vi "AlmacenamientoDatos.vi"(2 "array":dbl[](array[numeric])) -> ()   [LabVIEW 2014]
doc: "Demonstrates how to create a .xlsx file with the Write To Measurement File Express VI. A .xlsx file can be opened in Microsoft Excel 2007 or later. Running this example does not require Microsoft Excel to be installed on this computer."
panel:
  out "appended array":dbl[](array[numeric])
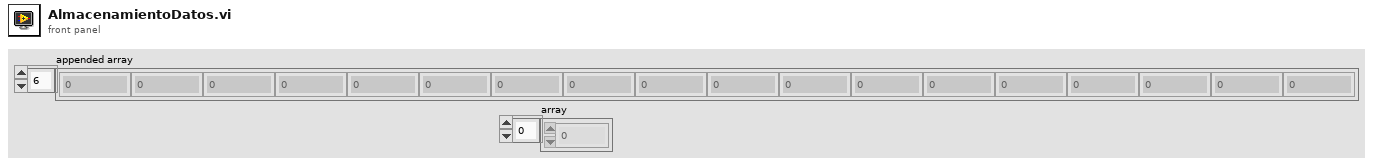
[diagram p1: front panel]
types:
  T1 = enum16{"big-endian, network order", "native, host order", "little-endian"}
  T2 = enum16{"open", "replace", "create", "open or create", "replace or create", "replace or create with confirmation"}
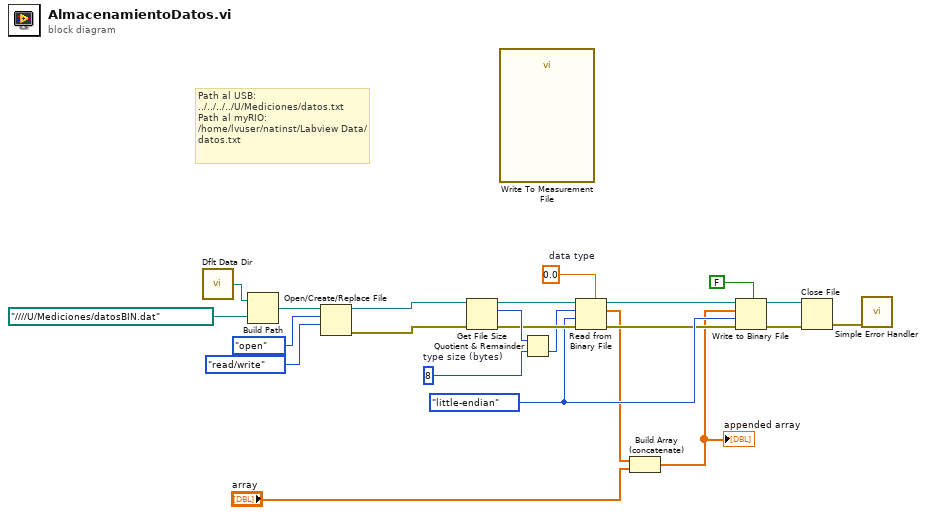
[diagram p0: block diagram]
diagram:
  w4 = 0.0  # data type
  w11 = i64 8  # type size (bytes)
  w8 = T1."little-endian" ("byte order (0:big-endian, network order)")
  # "Path al USB:\n../../../../U/Mediciones/datos.txt\nPath al myRIO:\n/home/lvuser/natinst/Labview Data/datos.txt"
  n1 = call <vilib>:"Dflt Data Dir.vi"() -> ("App:Default Data Directory"=w23:path)
  n2 = Build Path(base path=w23, name or relative path=path "../../../../U/Mediciones/datosBIN.dat" ("default name")) -> (appended path=w22:path)
  n3 = Open/Create/Replace File(file path (use dialog)=w22, operation (0:open)=T2."open", access (0:read/write)=enum16{"read/write", "read-only", "write-only"}."read/write") -> (refnum out=w13:refnum<file>, error out=w12:errorcluster)  [unwired: 1 in, 3 out]
  n4 = Get File Size(file=w13, error in=w12) -> (refnum out=w10:refnum<file>, size (in bytes)=w14:i64, 0:w9:errorcluster)
  n5 = call "Write To Measurement File"() -> ()  [unwired: 17 in, 3 out]
  n6 = Quotient & Remainder(x=w14, y=w11) -> (floor(x/y)=w7:i64)  [unwired: 1 out]
  n7 = Read from Binary File(5:w4, 8:w9, 9:w8, 10:w7, 11:w10) -> (0:w5:errorcluster, 2:w3:dbl[], 3:w6:refnum<file>)  [unwired: 1 in, 1 out]
  n8 = Build Array (concatenate)(w3, "array") -> (w1:dbl[])
  "appended array" <- w1
  n9 = Write to Binary File(file (use dialog)=w6, data=w1, error in=w5, 5:FALSE ("prepend array or string size? (T)"), 9:w8) -> (refnum out=w18:refnum<file>, error out=w19:errorcluster)  [unwired: 1 in, 1 out]
  n10 = Close File(refnum=w18, error in=w19) -> (error out=w21:errorcluster)  [unwired: 1 out]
  n11 = call <vilib>:"Simple Error Handler.vi"("error in (no error)"=w21) -> ()  [unwired: 1 in, 8 out]
